vi "FRCts20_Backend_Team_GET_reform.vi"(6 "eventdata":variant[][](array[variant]), 7 "Team":T1, 8 "error in (no error)":errorcluster, 10 "reqdata":variant[][](array[variant]), 11 "teamdata":variant[][](array[variant])) -> (0 "error out":errorcluster, 2 "data string":string)   [LabVIEW 2013, in "FRCts20_Backend_Engine.lvlib"]
doc: "Reforms and returns the specific team's data"
uses:
  FRCts20_Backend_Engine.lvlib
  FRCts20_Backend_API/FRCts20_Backend_API_Team.ctl
  FRCts20_Backend_API/FRCts20_Backend_API_SW.ctl
  FRCts20_Backend_API/FRCts20_Backend_API_Status.ctl
  FRCts20_Backend_DBCluster_TeamRoot_GET.ctl
  FRCts20_Backend_DBCluster_Team_GET_req.ctl
  <vilib>/addons/database/_DB Variant To Data/Database Variant To Data.xnode
  FRCts20_Backend_API/FRCts20_Backend_API.lvlib
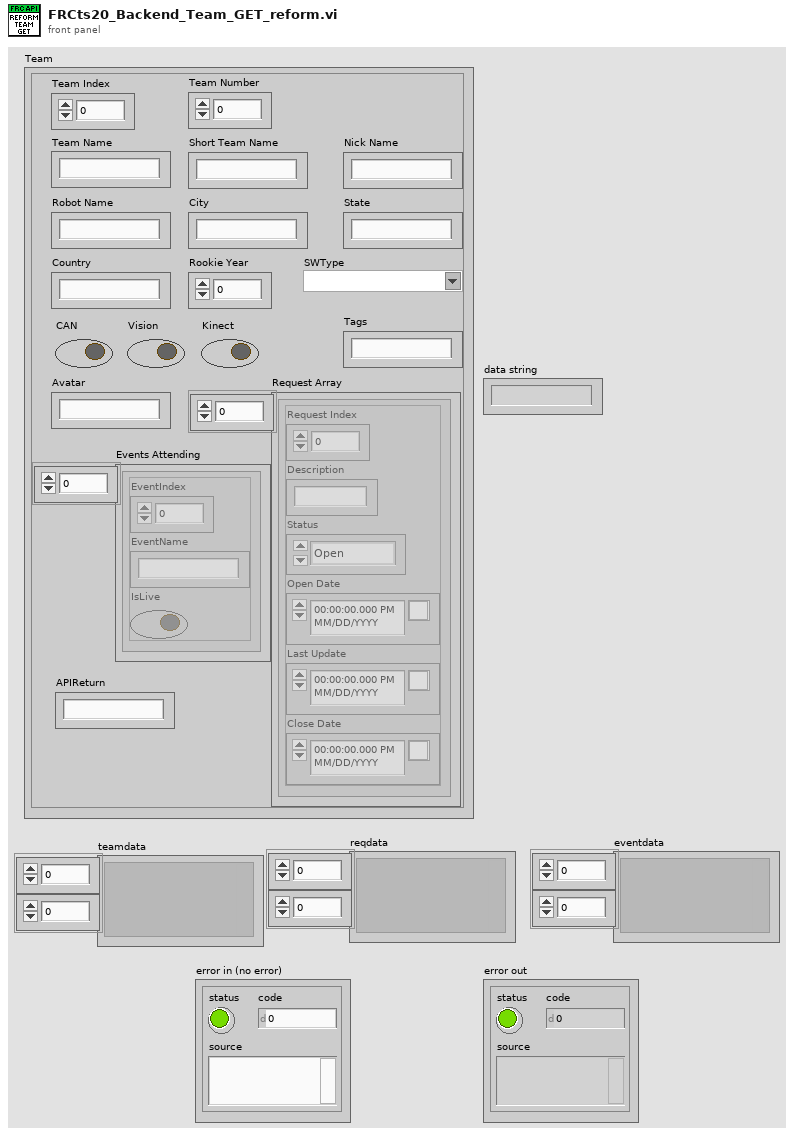
[diagram p1: front panel]
types:
  T1 = typedef "FRCts20_Backend_API.lvlib/FRCts20_Backend_API_Team.ctl" = cluster{"Team Index":u32, "Team Number":u32, "Team Name":string, "Short Team Name":string, "Nick Name":string, "Robot Name":string, "City":string, "State":string, "Country":string, "Rookie Year":u32, "SWType":T2, "CAN":bool, "Vision":bool, "Kinect":bool, "Tags":string, "Avatar":string, "Request Array":cluster{"Request Index":u32, "Description":string, "Status":T3, "Open Date":timestamp, "Last Update":timestamp, "Close Date":timestamp}[], "Events Attending":cluster{"EventIndex":dbl, "EventName":string, "IsLive":bool}[], "APIReturn":string}
  T2 = typedef "FRCts20_Backend_API.lvlib/FRCts20_Backend_API_SW.ctl" = string
  T3 = typedef "FRCts20_Backend_API.lvlib/FRCts20_Backend_API_Status.ctl" = enum16{"Open", "In Work", "Closed"}
  T4 = typedef "FRCts20_Backend_Engine.lvlib/FRCts20_Backend_DBCluster_Team_GET_req.ctl" = cluster{"ReqNumber":u32, "Description":string, "Status":T3, "OpenDate":timestamp, "LastUpdate":timestamp, "CloseDate":timestamp}
  T5 = typedef "FRCts20_Backend_Engine.lvlib/FRCts20_Backend_DBCluster_TeamRoot_GET.ctl" = cluster{"TeamIndex":u32, "TeamID":u32, "TeamNumber":u32, "TeamName":string, "ShortTeamName":string, "NickName":string, "RobotName":string, "City":string, "State":string, "Country":string, "Rookie Year":u32, "SWType":T2, "CAN":bool, "Vision":bool, "Kinect":bool, "Tags":string, "Avatar":string}
  T6 = cluster{"EventIndex":dbl, "EventName":string, "IsLive":bool}[]
  T7 = cluster{"Request Index":u32, "Description":string, "Status":T3, "Open Date":timestamp, "Last Update":timestamp, "Close Date":timestamp}[]
  T8 = cluster{"Request Index":u32, "Description":string, "Status":T3, "Open Date":timestamp, "Last Update":timestamp, "Close Date":timestamp}
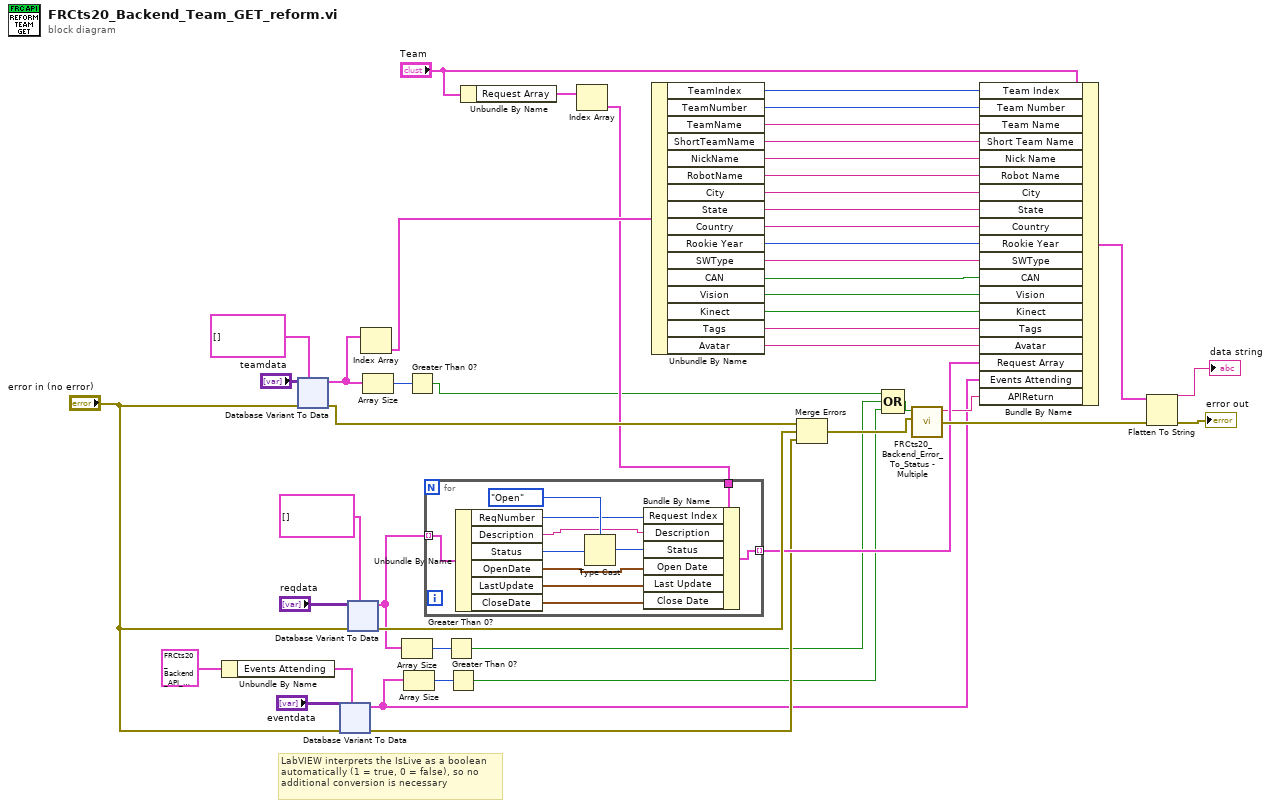
[diagram p0: block diagram]
diagram:
  # "LabVIEW interprets the IsLive as a boolean\nautomatically (1 = true, 0 = false), so no\nadditional conversion is necessary"
  n1 = Unbundle By Name(T1 {"Team Index"=0, "Team Number"=0, "Team Name"="", "Short Team Name"="", "Nick Name"="", "Robot Name"="", "City"="", "State"="", "Country"="", "Rookie Year"=0, "SWType"="", "CAN"=FALSE, "Vision"=FALSE, "Kinect"=FALSE, "Tags"="", "Avatar"="", "Request Array"=[], "Events Attending"=[], "APIReturn"=""} ("Team")) -> ("Events Attending"=w16:T6)
  n2 = xnode "Database Variant To Data"("database variant"="teamdata", "error in (no error)"="error in (no error)", "type"=T5[] []) -> ("data"=w38:T5[], "error out"=w40:errorcluster)
  n3 = xnode "Database Variant To Data"("database variant"="eventdata", "error in (no error)"="error in (no error)", "type"=w16) -> ("data"=w5:T6, "error out"=w14:errorcluster)
  n4 = xnode "Database Variant To Data"("database variant"="reqdata", "error in (no error)"="error in (no error)", "type"=T4[] []) -> ("data"=w7:T4[], "error out"=w39:errorcluster)
  n5 = Index Array(array=w38) -> (element=w25:T5)  [unwired: 1 in]
  n6 = Array Size(array=w38) -> (size(s)=w9:i32)
  n7 = Array Size(array=w7) -> (size(s)=w8:i32)
  n8 = Array Size(array=w5) -> (size(s)=w6:i32)
  n9 = Greater Than 0?(x=w9) -> (x > 0?=w2:bool)
  n10 = Greater Than 0?(x=w8) -> (x > 0?=w3:bool)
  n11 = Greater Than 0?(x=w6) -> (x > 0?=w4:bool)
  n12 = Unbundle By Name("Team") -> ("Request Array"=w23:T7)
  n13 = Index Array(array=w23) -> (element=w22:T8)  [unwired: 1 in]
  n14 = for {
    tunnel: w7 -> [w59] mode=indexing
    tunnel: w22 -> [w56]
    tunnel: [w50] -> w21 mode=indexing
    n15 = Unbundle By Name(w59) -> ("ReqNumber"=w55:u32, "Description"=w54:string, "Status"=w58:T3, "OpenDate"=w52:timestamp, "LastUpdate"=w51:timestamp, "CloseDate"=w49:timestamp)
    n16 = Type Cast(type=FRCts20_Backend_API_Status."Open" ("Status"), x=w58) -> (*(type *) &x=w53:T3)
    n17 = Bundle By Name(cluster=w56, "Request Index"=w55, "Description"=w54, "Status"=w53, "Open Date"=w52, "Last Update"=w51, "Close Date"=w49) -> (w50:T8)
  }
  n18 = Unbundle By Name(w25) -> ("TeamIndex"=w26:u32, "TeamNumber"=w37:u32, "TeamName"=w36:string, "ShortTeamName"=w35:string, "NickName"=w34:string, "RobotName"=w33:string, "City"=w32:string, "State"=w31:string, "Country"=w30:string, "Rookie Year"=w29:u32, "SWType"=w19:T2, "CAN"=w12:bool, "Vision"=w11:bool, "Kinect"=w10:bool, "Tags"=w28:string, "Avatar"=w27:string)
  n19 = Merge Errors(w40, w39, w14) -> (w41:errorcluster)
  n20 = Compound Arithmetic op=OR(w2, w3, w4) -> (w1:bool)
  n21 = call "FRCts20_Backend_Error_To_Status - Multiple.vi"("error in (no error)"=w41, "rows affected?"=w1) -> ("error out"=w47:errorcluster, "String"=w13:string)  [unwired: 8 in]
  n22 = Bundle By Name(cluster="Team", "Team Index"=w26, "Team Number"=w37, "Team Name"=w36, "Short Team Name"=w35, "Nick Name"=w34, "Robot Name"=w33, "City"=w32, "State"=w31, "Country"=w30, "Rookie Year"=w29, "SWType"=w19, "CAN"=w12, "Vision"=w11, "Kinect"=w10, "Tags"=w28, "Avatar"=w27, "Request Array"=w21, "Events Attending"=w5, "APIReturn"=w13) -> (w20:T1)
  n23 = Flatten To String(anything=w20, error in (no error)=w47) -> (data string=→"data string":string, error out=→"error out":errorcluster)  [unwired: 2 in, 1 out]
